vi "Loop Template.vi"() -> ()   [LabVIEW 2014]
uses:
  user.lib/_NEVSTOP/Communicable State Machine(CSM)/_Support/Priority Queue/Priority Queue.lvclass/Priority Queue.ctl
  user.lib/_NEVSTOP/Communicable State Machine(CSM)/_Support/Process/CSMP-Async Call.vi
  user.lib/_NEVSTOP/Communicable State Machine(CSM)/_Support/GlobalEvent/GEvt-Generate Status Log.vi
  user.lib/_NEVSTOP/Communicable State Machine(CSM)/_Support/Process/CSMP-Broadcast.vi
  user.lib/_NEVSTOP/Communicable State Machine(CSM)/_Support/GlobalEvent/GEvt-Generate Interrupt Log.vi
  user.lib/_NEVSTOP/Communicable State Machine(CSM)/_Support/GlobalEvent/GEvt-Generate Register Log.vi
  user.lib/_NEVSTOP/Communicable State Machine(CSM)/_Support/Process/CSMP-Register Status.vi
  user.lib/_NEVSTOP/Communicable State Machine(CSM)/_Support/GlobalEvent/GEvt-Generate Unregister Log.vi
  user.lib/_NEVSTOP/Communicable State Machine(CSM)/_Support/Process/CSMP-Unregister Status.vi
  user.lib/_NEVSTOP/Communicable State Machine(CSM)/_Support/Process/CSMP-Sync Call.vi
  user.lib/_NEVSTOP/Communicable State Machine(CSM)/_Support/CSMQ/_CSMObj-Unlock.vi
  user.lib/_NEVSTOP/Communicable State Machine(CSM)/_Support/Process/CSMP-PostPostMsg.vi
  user.lib/_NEVSTOP/Communicable State Machine(CSM)/_Support/Process/CSMP-PostSendMsg.vi
  user.lib/_NEVSTOP/Communicable State Machine(CSM)/_Support/CSMQ/_CSMObj-Lock State.vi
  user.lib/_NEVSTOP/Communicable State Machine(CSM)/_Support/Common/Splite Reason String Part.vi
  user.lib/_NEVSTOP/Communicable State Machine(CSM)/_Support/Common/Trim Single line Text.vi
  user.lib/_NEVSTOP/Communicable State Machine(CSM)/_Support/CSMQ/_CSMOFGV Release.vi
  user.lib/_NEVSTOP/Communicable State Machine(CSM)/_Support/Common/Remove Comments from Line.vi
  user.lib/_NEVSTOP/Communicable State Machine(CSM)/_Support/Common/Splite Single-line Message.vi
  user.lib/_NEVSTOP/Communicable State Machine(CSM)/_Support/Common/Parse Next Single-line State.vi
  user.lib/_NEVSTOP/Communicable State Machine(CSM)/_Support/CSMQ/_CSMOFGV Dequeue.vi
  user.lib/_NEVSTOP/Communicable State Machine(CSM)/_Support/CSMQ/_CSMObj-Log Error if in a Remote Session.vi
  user.lib/_NEVSTOP/Communicable State Machine(CSM)/_Support/GlobalEvent/GEvt-Generate State Change Log.vi
  user.lib/_NEVSTOP/Communicable State Machine(CSM)/_Support/GlobalEvent/GEvt-Generate Remaining States Log.vi
  user.lib/_NEVSTOP/Communicable State Machine(CSM)/_Support/GlobalEvent/GEvt-Generate Module Destroyed Log.vi
  user.lib/_NEVSTOP/Communicable State Machine(CSM)/_Support/GlobalEvent/GEvt-Generate Complete Log.vi
  user.lib/_NEVSTOP/Communicable State Machine(CSM)/_Support/GlobalEvent/GEvt-Generate Module Created Log.vi
  user.lib/_NEVSTOP/Communicable State Machine(CSM)/AdvanceAPI/CSM - Revert Arguments-Safe String.vi
  user.lib/_NEVSTOP/Communicable State Machine(CSM)/AdvanceAPI/CSM - Make String Arguments Safe.vi
  user.lib/_NEVSTOP/Communicable State Machine(CSM)/_Support/CSMQ/_CSMObj-Message Check.vi
  user.lib/_NEVSTOP/Communicable State Machine(CSM)/_Support/CSMQ/_CSMObj-Enqueue Cross-Module Message.vi
  user.lib/_NEVSTOP/Communicable State Machine(CSM)/_Support/CSMQ/_CSMOFGV Get.vi
  user.lib/_NEVSTOP/Communicable State Machine(CSM)/_Support/FGV-BroadcastRegistry/Cache-Broadcast Registry Search Result.vi
  user.lib/_NEVSTOP/Communicable State Machine(CSM)/AdvanceAPI/CSM - Register Status Change.vi
  user.lib/_NEVSTOP/Communicable State Machine(CSM)/AdvanceAPI/CSM - Unregister Status Change.vi
  user.lib/_NEVSTOP/Communicable State Machine(CSM)/_Support/Common/Hex Str to U8 Data.vi
  user.lib/_NEVSTOP/Communicable State Machine(CSM)/_Support/Common/Concatenate State with Arguments.vi
  user.lib/_NEVSTOP/Communicable State Machine(CSM)/_Support/Common/U8 Data to Hex Str.vi
  user.lib/_NEVSTOP/Communicable State Machine(CSM)/_Support/Priority Queue/Dequeue Element.vi
  user.lib/_NEVSTOP/Communicable State Machine(CSM)/AdvanceAPI/CSM - Keywords.vi
  user.lib/_NEVSTOP/Communicable State Machine(CSM)/_Support/Priority Queue/Enqueue Element.vi
  user.lib/_NEVSTOP/Communicable State Machine(CSM)/Utility/Trim Both Whitespace.vi
  user.lib/_NEVSTOP/Communicable State Machine(CSM)/_Support/GlobalEvent/FGV-GlobalEventRef.vi
  user.lib/_NEVSTOP/Communicable State Machine(CSM)/_Support/CSMQ/_CSMOFGV Obtain.vi
  user.lib/_NEVSTOP/Communicable State Machine(CSM)/_Support/CSMQ/_CSMOFGV.vi
  user.lib/_NEVSTOP/Communicable State Machine(CSM)/_Support/GlobalEvent/FGV-StatusChangeEventRef.vi
  user.lib/_NEVSTOP/Communicable State Machine(CSM)/_Support/FGV-BroadcastRegistry/global-Broadcast Cache Change Flag.vi
  user.lib/_NEVSTOP/Communicable State Machine(CSM)/_Support/FGV-BroadcastRegistry/FGV-BroadcastRegistry.vi
  user.lib/_NEVSTOP/Communicable State Machine(CSM)/Communicable State Machine.lvlib
  user.lib/_NEVSTOP/Communicable State Machine(CSM)/addons/Loop-Support/CSM Loop Support.lvlib
panel:
  out "Filtered UI States":string
  out "UI States":string
  out ">> Source CSM >>":string
  out "Remaining States":string
  in  "DAQ: Once":bool
  out "Waveform Chart":dbl(graph)=7.7472539242125515
  in  "Center":dbl(slide) scale=0.0..10.0
  in  "Stop":bool
  in  "Start":bool
  out "State History":string
  in  "Name(\"\" to use uuid)":string="CSM Tiny"
  in  "Init State(\"Macro: Initialize\")":string="Macro: Initialize"
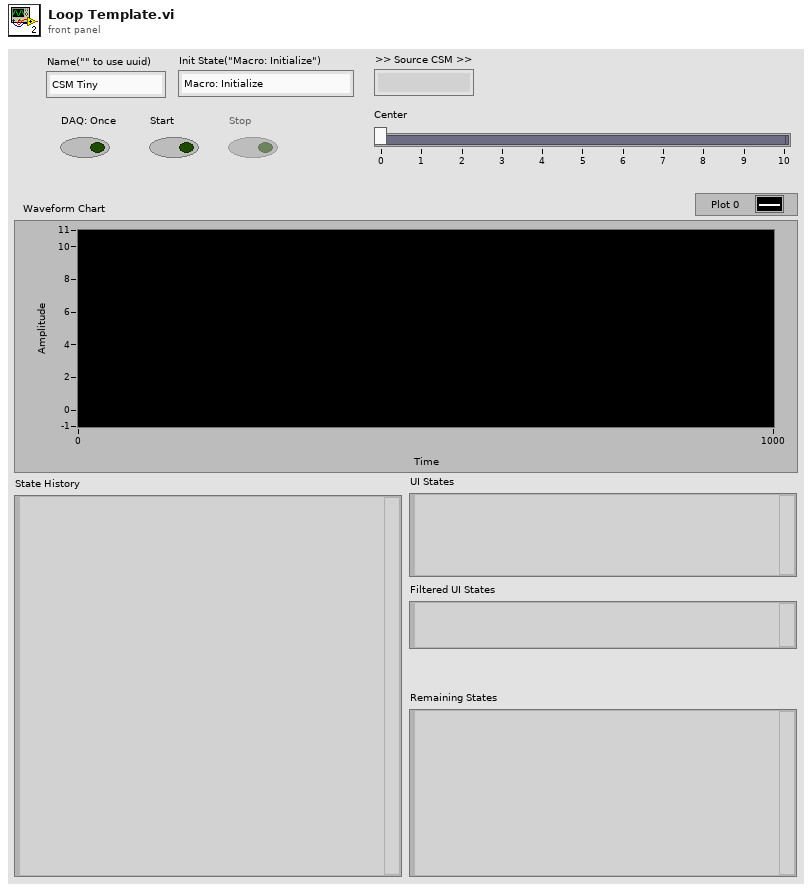
[diagram p1: front panel]
types:
  T1 = enum32{"Invalid", "Standard", "Closed", "Hidden", "Minimized", "Maximized"}
  T2 = enum32{"invalid app kind", "Development System", "Run Time System", "Student Edition", "Embedded LabVIEW", "Evaluation", "Custom"}
  T3 = typedef "Communicable State Machine.lvlib/_CSM_Response Source Message.ctl" = cluster{"‘State":string, "’Arguments":string, "’Error":errorcluster}
  T4 = cluster{"Core":cluster{"Current VI Reference":refnum<vi>, "Close Panel on Exit?":bool}, "IsRunning?":bool, "Center":dbl}
  T5 = cluster{"Current VI Reference":refnum<vi>, "Close Panel on Exit?":bool}
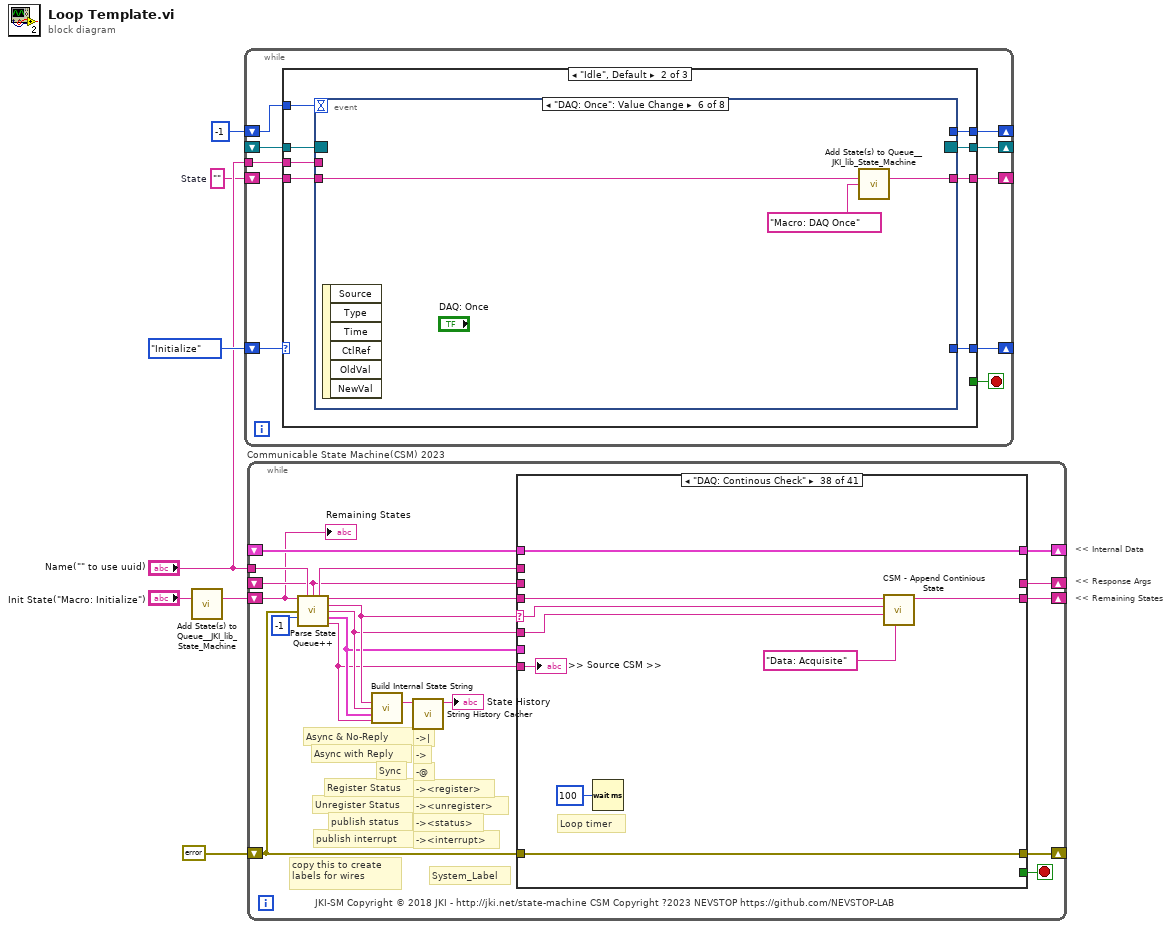
[diagram p0: block diagram]
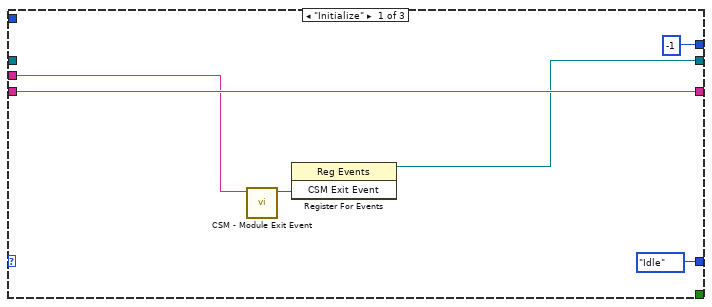
[diagram p2: hidden frame]
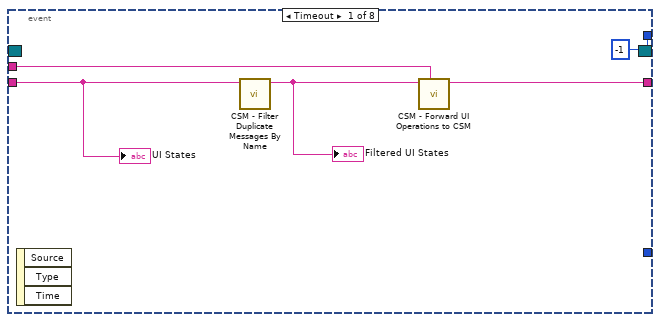
[diagram p3: hidden frame]
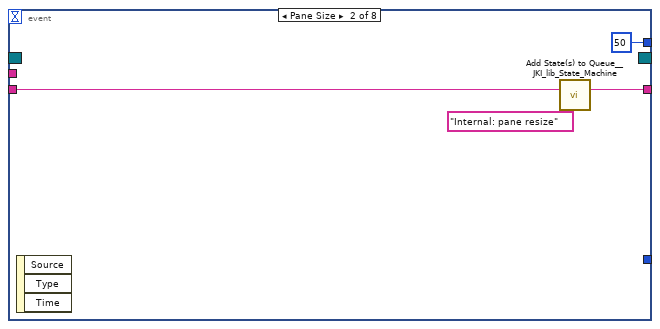
[diagram p4: hidden frame]
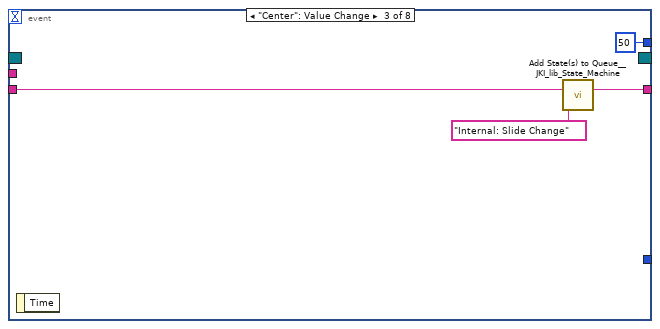
[diagram p5: hidden frame]
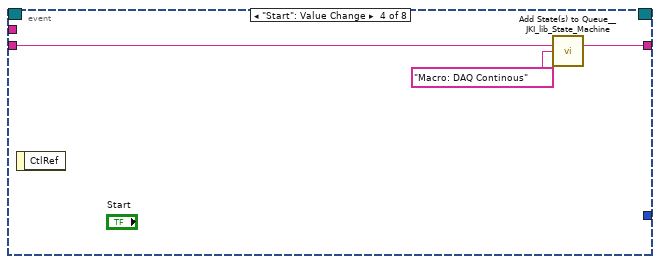
[diagram p6: hidden frame]
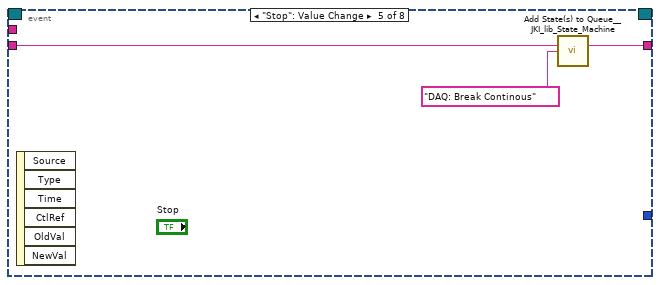
[diagram p7: hidden frame]
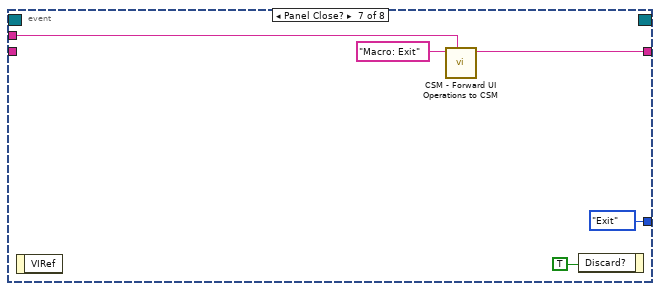
[diagram p8: hidden frame]
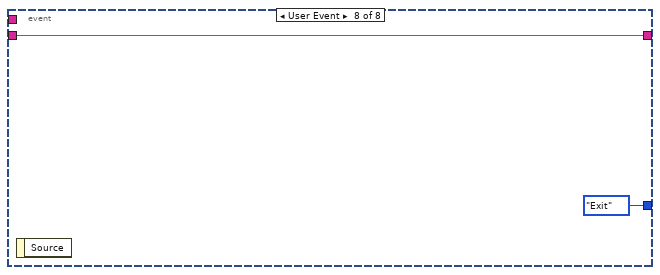
[diagram p9: hidden frame]
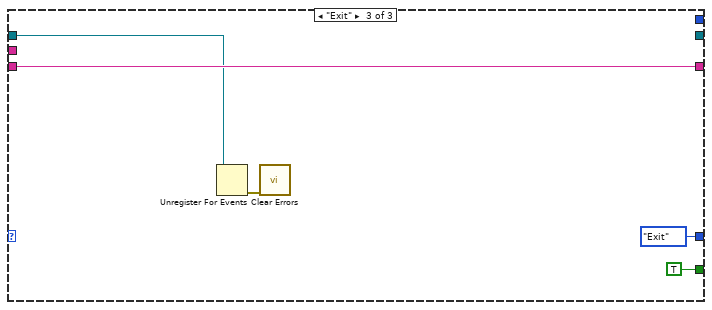
[diagram p10: hidden frame]
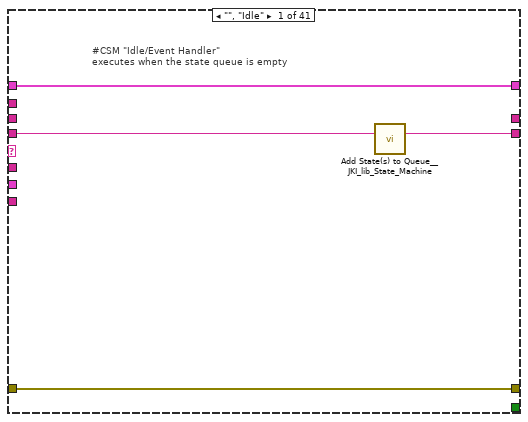
[diagram p11: hidden frame]
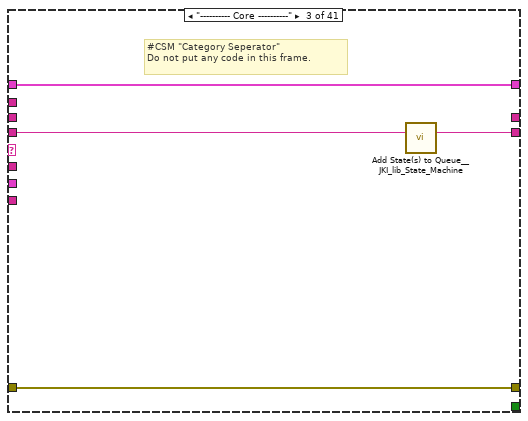
[diagram p13: hidden frame]
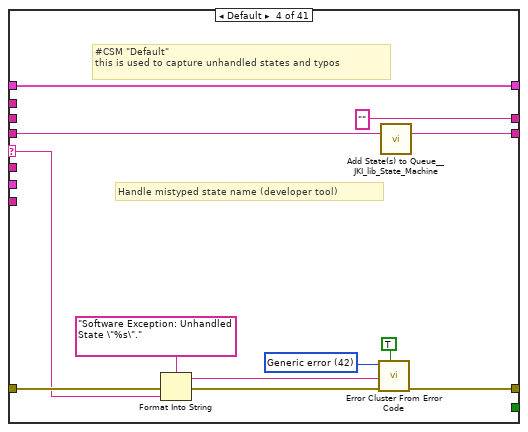
[diagram p14: hidden frame]
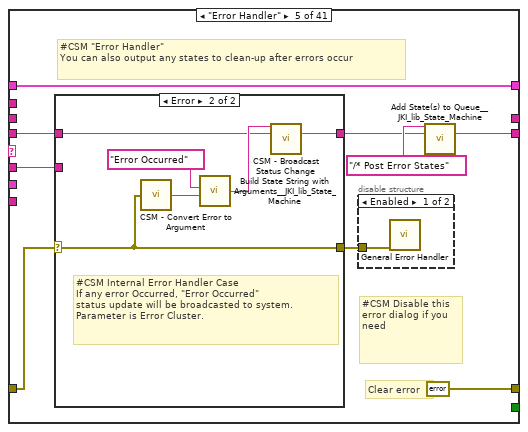
[diagram p15: hidden frame]
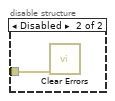
[diagram p16: hidden frame]
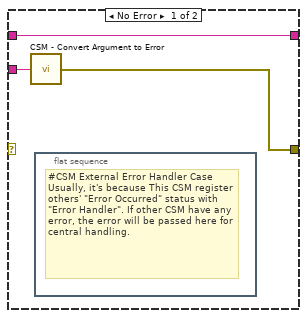
[diagram p17: hidden frame]
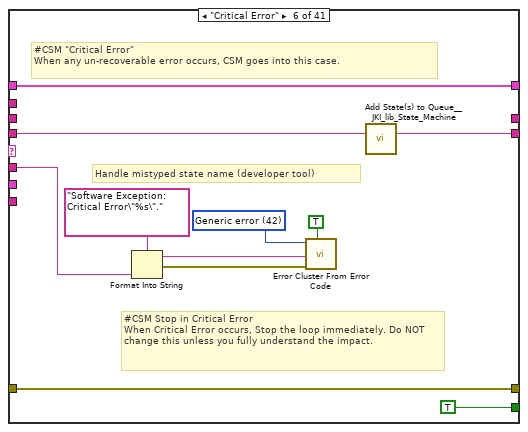
[diagram p18: hidden frame]
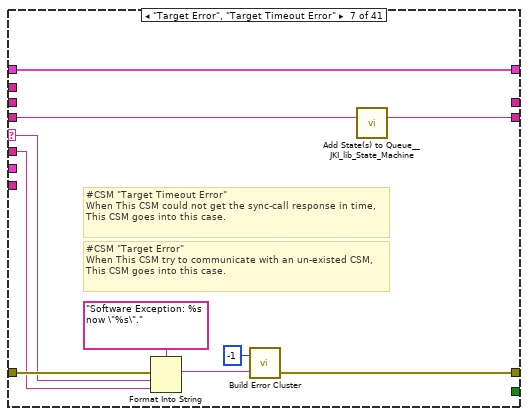
[diagram p19: hidden frame]
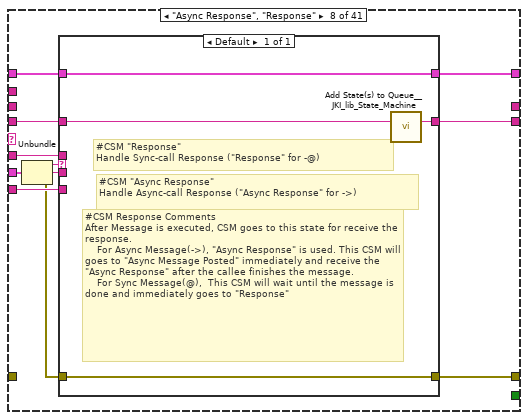
[diagram p20: hidden frame]
diagram:
  w2 = ""  # State
  # "<< Internal Data"
  # "<< Response Args"
  # "<< Remaining States"
  n1 = call <vilib>:"Add State(s) to Queue__JKI_lib_State_Machine.vi"("State(s) in (\"\")"="Init State(\"Macro: Initialize\")") -> ("States Out"=w5:string)  [unwired: 14 in]
  n2 = while {
    shift-right: [w16] -> _
    shift-left: enum16{"Idle", "Initialize", "Exit"}."Initialize" -> [w17]
    tunnel: "Name(\"\" to use uuid)" -> [w14]
    shift-right: [w12] -> _
    shift-left: w2 -> [w13]
    shift-right: [w10] -> _
    shift-left: -1 -> [w11]
    shift-right: [w9] -> _
    shift-left: _ -> [w8]
    stop <- w15 stop-if-true
    n3 = case shown="\"Idle\", Default" w17 {
      tunnel: [enum16{"Idle", "Initialize", "Exit"}."Idle" w31 enum16{"Idle", "Initialize", "Exit"}."Exit"] -> w16
      tunnel: [_ _ TRUE] -> w15
      tunnel: w14 -> [w19 w30 _]
      tunnel: w13 -> [w22 w28 w63]
      tunnel: [w22 w29 w63] -> w12
      tunnel: w11 -> [_ w26 _]
      tunnel: [-1 w27 _] -> w10
      tunnel: [w18 w24 _] -> w9
      tunnel: w8 -> [_ w25 w62]
      frame "Initialize" {
        n4 = call "CSM - Module Exit Event.vi"("Name(\"\" to use uuid) in"=w19) -> ("CSM Exit Event"=w20:refnum<user-event>)  [unwired: 9 in, 1 out]
        n5 = register-events(w20) -> (reference out=w18:refnum<event-registration>)  [unwired: 2 in, 1 out]
      }
      frame "Idle", Default {
        n6 = event shown="[5] \"DAQ: Once\": Value Change" {
          selector: w25 -> [_ _ _ _ _ _ _ _]
          dyn-events: [_ _ _ _ _ _ _ _] -> w24
          timeout: w26 -> [_ _ _ _ _ _ _ _]
          tunnel: [_ _ _ _ _ _ enum16{"Idle", "Initialize", "Exit"}."Exit" enum16{"Idle", "Initialize", "Exit"}."Exit"] -> w31
          tunnel: w30 -> [w32 _ _ _ _ _ w55 _]
          tunnel: w28 -> [w35 w40 w44 w47 w49 w52 _ w60]
          tunnel: [w33 w39 w43 w46 w50 w53 w54 w60] -> w29
          tunnel: [-1 50 50 _ _ _ _ _] -> w27
          event Timeout {
            n7 = event-data() -> ()  [unwired: 1 in, 3 out]
            n8 = call "CSM - Filter Duplicate Messages By Name.vi"("States"=w35) -> ("States out"=w34:string)  [unwired: 10 in]
            "Filtered UI States" <- w34
            n9 = call "CSM - Forward UI Operations to CSM.vi"("Name(\"\" to use uuid)"=w32, "State(s) in (\"\")"=w34) -> ("States Out"=w33:string)  [unwired: 9 in]
            "UI States" <- w35
          }
          event Pane Size {
            n10 = event-data() -> ()  [unwired: 1 in, 3 out]
            n11 = call <vilib>:"Add State(s) to Queue__JKI_lib_State_Machine.vi"("State(s) in (\"\")"=w40, "State(s) at Back (\"\")"="Internal: pane resize" ("State(s) at Back (\"\")")) -> ("States Out"=w39:string)  [unwired: 13 in]
          }
          event "Center": Value Change {
            n12 = event-data() -> ()  [unwired: 1 in, 1 out]
            n13 = call <vilib>:"Add State(s) to Queue__JKI_lib_State_Machine.vi"("State(s) in (\"\")"=w44, "State(s) at Back (\"\")"="Internal: Slide Change" ("State(s) at Back (\"\")")) -> ("States Out"=w43:string)  [unwired: 13 in]
          }
          event "Start": Value Change {
            n14 = event-data() -> ()  [unwired: 1 in, 1 out]
            n15 = call <vilib>:"Add State(s) to Queue__JKI_lib_State_Machine.vi"("State(s) in (\"\")"=w47, "State(s) at Back (\"\")"="Macro: DAQ Continous" ("State(s) at Back (\"\")")) -> ("States Out"=w46:string)  [unwired: 13 in]
          }
          event "Stop": Value Change {
            n16 = event-data() -> ()  [unwired: 1 in, 6 out]
            n17 = call <vilib>:"Add State(s) to Queue__JKI_lib_State_Machine.vi"("State(s) in (\"\")"=w49, "State(s) at Back (\"\")"="DAQ: Break Continous" ("State(s) at Back (\"\")")) -> ("States Out"=w50:string)  [unwired: 13 in]
          }
          event "DAQ: Once": Value Change {
            n18 = event-data() -> ()  [unwired: 1 in, 6 out]
            n19 = call <vilib>:"Add State(s) to Queue__JKI_lib_State_Machine.vi"("State(s) in (\"\")"=w52, "State(s) at Back (\"\")"="Macro: DAQ Once" ("State(s) at Back (\"\")")) -> ("States Out"=w53:string)  [unwired: 13 in]
          }
          event Panel Close? {
            n20 = event-data() -> ()  [unwired: 1 in, 1 out]
            n21 = call "CSM - Forward UI Operations to CSM.vi"("Name(\"\" to use uuid)"=w55, "State(s) in (\"\")"="Macro: Exit" ("State")) -> ("States Out"=w54:string)  [unwired: 9 in]
            n22 = event-data("Discard?"=TRUE) -> ()  [unwired: 1 in, 1 out]
          }
          event User Event {
            n23 = event-data() -> ()  [unwired: 1 in, 1 out]
          }
        }
      }
      frame "Exit" {
        n24 = Unregister For Events(event registration refnum=w62) -> (error out=w61:errorcluster)  [unwired: 1 in]
        n25 = call <vilib>:"Clear Errors.vi"("error in (no error)"=w61) -> ()  [unwired: 5 in, 2 out]
      }
    }
  }
  n26 = while "Communicable State Machine(CSM) 2023" {
    shift-right: [w80] -> _
    shift-left: _ -> [w79]
    shift-right: [w83] -> _
    shift-left: errorcluster {"status"=FALSE, "code"=0, "source"=""} ("error out") -> [w78]
    shift-right: [w82] -> _
    shift-left: w5 -> [w66]
    tunnel: "Name(\"\" to use uuid)" -> [w76]
    shift-right: [w77] -> _
    shift-left: _ -> [w68]
    stop <- w81 stop-if-true
    # "-><interrupt>"
    # "-><status>"
    # "-><unregister>"
    # "-><register>"
    # "-@"
    # "->"
    # "->|"
    # "publish interrupt"
    # "publish status"
    # "Unregister Status"
    # "Register Status"
    # "Sync"
    # "Async with Reply"
    # "Async & No-Reply"
    # "copy this to create labels for wires"
    # "System_Label"
    # "JKI-SM Copyright © 2018 JKI - http://jki.net/state-machine CSM Copyright ?2023 NEVSTOP https://github.com/NEVSTOP-LAB"
    n27 = call "Parse State Queue++.vi"("State Queue"=w66, "Name(\"\" to use uuid)"=w76, "Response Arguments"=w68, "Error In (no error)"=w78, "Dequeue Timeout(0ms)"=-1 ("Timeout")) -> ("Name Used"=w69:string, "Remaining States"=w84:string, "Current State"=w73:string, "Arguments"=w72:string, ">> Response Source Message >>"=w71:T3, ">> Source CSM >>"=w70:string)  [unwired: 5 in]
    n28 = call "Build Internal State String.vi"("State"=w73, "Arguments (\"\")"=w72, ">> Response Source Message >>"=w71, "Source (\"\")"=w70) -> ("State with Arguments"=w74:string)  [unwired: 11 in]
    n29 = call "String History Cacher.vi"("String"=w74) -> ("String Cache"=→"State History":string)  [unwired: 10 in]
    n30 = case shown="\"DAQ: Continous Check\"" w73 {
      selector: w73 -> [_ _ _ w97 _ _ w142 _ _ _ _ _ _ _ _ _ _ _ _ _ _ _ _ _ _ _ _ _ _ _ _ _ _ _ _ _ _ w394 _ _ _]
      tunnel: w84 -> [w85 w90 w95 w101 w112 w136 w144 w154 w165 w179 w184 w188 w195 w197 w204 w208 w214 w220 w235 w313 w318 w323 w325 w330 w334 w342 w346 w351 w358 w362 w366 w370 w373 w376 w379 w384 w390 w396 w402 w408 w411]
      tunnel: w72 -> [_ _ _ _ w111 w129 w143 w153 _ _ _ _ _ _ _ _ _ w215 w229 _ _ _ _ _ _ _ _ w349 _ _ _ _ _ _ _ _ _ w393 _ _ _]
      tunnel: w79 -> [w86 w89 w92 w99 w115 w137 w145 w156 w164 w172 w182 w185 _ w196 w199 w205 w212 w218 w231 w312 w315 w320 w327 w332 w336 w341 w345 w350 w355 w359 w363 w369 w372 w375 w378 w383 w387 w399 w403 w407 w410]
      tunnel: [w87 w91 w93 w103 errorcluster {"status"=FALSE, "code"=0, "source"=""} ("error out") w138 w140 w159 w166 w176 w181 w186 w192 w198 w200 w206 w211 w216 w232 w314 w316 w321 w328 w333 w339 w343 w347 w352 w356 w360 w364 w371 w374 w377 w380 w385 w391 w400 w404 w409 w412] -> w83
      tunnel: w78 -> [w87 w91 w93 w102 w113 w138 w147 _ w166 w176 w181 w186 w192 w198 w201 w206 w211 w217 w233 w314 w316 w321 w328 w333 w339 w343 w347 w352 w356 w360 w364 w371 w374 w377 w380 w385 w391 w400 w404 w409 w412]
      tunnel: [w88 w90 w94 w100 w108 w135 w146 w155 w165 w178 w183 w187 w194 w197 w203 w207 w213 w219 w234 w313 w317 w322 w326 w331 w340 w342 w346 w351 w357 w361 w365 w370 w373 w376 w379 w384 w390 w397 w401 w408 w411] -> w82
      tunnel: [_ _ _ _ _ TRUE _ _ _ _ TRUE _ _ _ _ _ _ _ _ _ _ _ _ _ _ _ _ _ _ _ _ _ _ _ _ _ _ _ _ _ _] -> w81
      tunnel: [w86 w89 w92 w99 w115 w137 w145 w157 w164 w177 w182 w185 w193 w196 w199 w205 w212 w218 w231 w312 w315 w320 w327 w332 w336 w341 w345 w350 w355 w359 w363 w368 w372 w375 w378 w382 w387 w399 w403 w406 w410] -> w80
      tunnel: w70 -> [_ _ _ _ _ _ _ w151 _ _ _ _ _ _ _ _ _ _ _ _ _ _ _ _ _ _ _ _ _ _ _ _ _ _ _ _ _ w395 _ _ _]
      tunnel: w71 -> [_ _ _ _ _ _ _ w158 _ _ _ _ _ _ _ _ _ _ _ _ _ _ _ _ _ _ _ _ _ _ _ _ _ _ _ _ _ _ _ _ _]
      tunnel: [_ _ _ "" _ _ _ _ _ _ _ _ _ _ _ _ _ _ _ _ _ _ _ _ _ _ "API1 Response" w348 _ _ _ _ _ _ _ _ _ _ _ _ _] -> w77
      tunnel: w69 -> [_ _ _ _ _ _ _ _ _ _ _ _ _ _ _ _ _ _ _ _ _ _ _ _ _ _ _ _ _ _ _ _ _ _ _ _ _ _ _ _ _]
      tunnel: w68 -> [_ _ _ _ _ _ _ _ _ _ _ _ _ _ _ _ _ _ _ _ _ _ _ _ _ _ _ _ _ _ _ _ _ _ _ _ _ _ _ _ _]
      frame "", "Idle" {
        # "#CSM \"Idle/Event Handler\"\nexecutes when the state queue is empty"
        n31 = call <vilib>:"Add State(s) to Queue__JKI_lib_State_Machine.vi"("State(s) in (\"\")"=w85) -> ("States Out"=w88:string)  [unwired: 14 in]
      }
      frame "CSM Documentation" {
        # "#CSM README FIRST\n\nCSM is a LabVIEW application framework that builds upon JKI State Machine (JKISM). It follows the pattern of JKISM and extends the keywords to describe message communication between CSM modules, including concepts such as Sync-Message, Async-Message, Subscription/Unsubscription of status - essential elements for creating reusable code modules. For more information, please visit the CSM wiki: https://github.com/NEVSTOP-LAB/JKI-State-Machine-Plus-Plus/wiki\n\nFor instructions on JKI State Machine, visit: http://jki.net/state-machine/\nFor information about CSM, visit: https://github.com/NEVSTOP-LAB"
        # "#CSM \"Documentation\"\nCase for holding CSM Documenation"
      }
      frame "---------- Core ----------" {
        # "#CSM \"Category Seperator\"\nDo not put any code in this frame."
        n32 = call <vilib>:"Add State(s) to Queue__JKI_lib_State_Machine.vi"("State(s) in (\"\")"=w95) -> ("States Out"=w94:string)  [unwired: 14 in]
      }
      frame Default {
        w106 = 42 items=["No error", "Argument error", "Memory is full", "Out of zone", "End of file", "File already open", "Generic file I/O error", "File not found", "File permission error", "Disk is full", "Duplicate path", "Too many files open", "System feature not enabled", "Resource file not found", "Cannot add resource", "Resource not found", "Image not found", "Image memory error", "Pen does not exist", "Config type invalid", "Config token not found", "Config parse error", "Config memory error", "Bad external code format", "Bad external code offset", "External code not present", "Null window", "Destroy window error", "Null menu", "Print aborted", "Bad print record", "Print driver error", "Windows error during printing", "Memory error during printing", "Print dialog error", "Generic print error", "Invalid device refnum", "Device not found", "Device parameter error", "Device unit error", "Cannot open device", "Device call aborted", "Generic error", "Cancelled by user", "Object ID too low", "Object ID too high", "Object not in heap", "Unknown heap", "Unknown object (invalid DefProc)", "Unknown object (DefProc not in table)", "Message out of range", "Invalid (null) method", "Unknown message", "Manager call not supported", "Bad address", "Network operation in progress", "Network operation timed out", "Connection is busy", "Network attribute not supported", "Network error", "Address in use", "System out of memory", "Connection aborted", "Connection refused", "Not connected", "Already connected", "Connection closed", "Initialization error (interapplication manager)", "Bad occurrence", "Wait on unbound occurrence handler", "Occurrence queue overflow", "Datalog type conflict", "Unused", "Unrecognized type (interapplication manager)", "Memory corrupt", "Failed to make temporary DLL", "Old CIN version", "Drag socket not found", "Failed to load drop-object", "Failed to register OLE object", "Failed to release OLE object", "Format specifier type mismatch", "Unknown format specifier", "Too few format specifiers", "Too many format specifiers", "Scan failed", "Newer CIN version", "Error converting to variant", "Runtime menu error", "Password tampered", "Variant attribute not found", "Incompatible variant data type", "Event data is not available", "Event Store is not present", "Occurrence is not found", "Event Queue is not created", "Event info is not available", "Refnum passed is NULL", "Error retrieving Class GUID", "Error retrieving CoClass GUID", "Error retrieving TypeLib GUID.", "Bad built application magic bytes.", "Specific driver is different from the specific driver associated with the Logical Name.", "There is no session opened to the class driver.", "Max Error", "MAX - Error with config objects", "MAX - Error loading configuration", "MAX - Group not supported"]
        # "#CSM \"Default\"\nthis is used to capture unhandled states and typos"
        # "Handle mistyped state name (developer tool)"
        n33 = Format Into String(format string="Software Exception: Unhandled State \"%s\"." ("message"), error in=w102, w97) -> (resulting string=w105:string, error out=w104:errorcluster)  [unwired: 1 in]
        n34 = call <vilib>:"Error Cluster From Error Code.vi"("show call chain? (False)"=TRUE, "error in (no error)"=w104, "error message (\"\")"=w105, "error code (0)"=w106) -> ("error out"=w103:errorcluster)  [unwired: 5 in]
        n35 = call <vilib>:"Add State(s) to Queue__JKI_lib_State_Machine.vi"("State(s) in (\"\")"=w101) -> ("States Out"=w100:string)  [unwired: 14 in]
      }
      frame "Error Handler" {
        # "#CSM Disable this error dialog if you need"
        # "#CSM \"Error Handler\"\nYou can also output any states to clean-up after errors occur"
        # "Clear error"
        n36 = case shown="Error" w113 {
          selector: w113 -> [_ w122]
          tunnel: [w121 w124] -> w109
          tunnel: w112 -> [w121 w123]
          tunnel: w111 -> [w120 _]
          tunnel: [w119 w122] -> w114
          frame No Error {
            n37 = call "CSM - Convert Argument to Error.vi"("Argument"=w120) -> ("error"=w119:errorcluster)  [unwired: 4 in]
            n38 = flat-sequence {
              frame #0 {
                # "#CSM External Error Handler Case\nUsually, it's because This CSM register others' \"Error Occurred\" status with \"Error Handler\". If other CSM have any error, the error will be passed here for central handling."
              }
            }
          }
          frame Error {
            # "#CSM Internal Error Handler Case \nIf any error Occurred, \"Error Occurred\" \nstatus update will be broadcasted to system.\nParameter is Error Cluster."
            n39 = call "CSM - Convert Error to Argument.vi"("error in (no error)"=w122) -> ("Arguments"=w126:string)  [unwired: 4 in]
            n40 = call <vilib>:"Build State String with Arguments__JKI_lib_State_Machine.vi"("Arguments (\"\")"=w126, "State"="Error Occurred" ("Status with Arguments")) -> ("State with Arguments"=w125:string)  [unwired: 4 in]
            n41 = call "CSM - Broadcast Status Change.vi"("Status with Arguments"=w125, "State Queue"=w123) -> ("Remaining States"=w124:string)  [unwired: 13 in]
          }
        }
        n42 = disable-structure shown="Enabled" {
          disable-tunnel: w114 -> [w117 w118]
          frame Enabled {
            n43 = call <vilib>:"General Error Handler.vi"("error in (no error)"=w117) -> ()  [unwired: 10 in, 5 out]
          }
          frame Disabled {
            n44 = call <vilib>:"Clear Errors.vi"("error in (no error)"=w118) -> ()  [unwired: 5 in, 2 out]
          }
        }
        n45 = call <vilib>:"Add State(s) to Queue__JKI_lib_State_Machine.vi"("State(s) in Front (\"\")"="/* Post Error States", "State(s) in (\"\")"=w109) -> ("States Out"=w108:string)  [unwired: 13 in]
      }
      frame "Critical Error" {
        w133 = 42 items=["No error", "Argument error", "Memory is full", "Out of zone", "End of file", "File already open", "Generic file I/O error", "File not found", "File permission error", "Disk is full", "Duplicate path", "Too many files open", "System feature not enabled", "Resource file not found", "Cannot add resource", "Resource not found", "Image not found", "Image memory error", "Pen does not exist", "Config type invalid", "Config token not found", "Config parse error", "Config memory error", "Bad external code format", "Bad external code offset", "External code not present", "Null window", "Destroy window error", "Null menu", "Print aborted", "Bad print record", "Print driver error", "Windows error during printing", "Memory error during printing", "Print dialog error", "Generic print error", "Invalid device refnum", "Device not found", "Device parameter error", "Device unit error", "Cannot open device", "Device call aborted", "Generic error", "Cancelled by user", "Object ID too low", "Object ID too high", "Object not in heap", "Unknown heap", "Unknown object (invalid DefProc)", "Unknown object (DefProc not in table)", "Message out of range", "Invalid (null) method", "Unknown message", "Manager call not supported", "Bad address", "Network operation in progress", "Network operation timed out", "Connection is busy", "Network attribute not supported", "Network error", "Address in use", "System out of memory", "Connection aborted", "Connection refused", "Not connected", "Already connected", "Connection closed", "Initialization error (interapplication manager)", "Bad occurrence", "Wait on unbound occurrence handler", "Occurrence queue overflow", "Datalog type conflict", "Unused", "Unrecognized type (interapplication manager)", "Memory corrupt", "Failed to make temporary DLL", "Old CIN version", "Drag socket not found", "Failed to load drop-object", "Failed to register OLE object", "Failed to release OLE object", "Format specifier type mismatch", "Unknown format specifier", "Too few format specifiers", "Too many format specifiers", "Scan failed", "Newer CIN version", "Error converting to variant", "Runtime menu error", "Password tampered", "Variant attribute not found", "Incompatible variant data type", "Event data is not available", "Event Store is not present", "Occurrence is not found", "Event Queue is not created", "Event info is not available", "Refnum passed is NULL", "Error retrieving Class GUID", "Error retrieving CoClass GUID", "Error retrieving TypeLib GUID.", "Bad built application magic bytes.", "Specific driver is different from the specific driver associated with the Logical Name.", "There is no session opened to the class driver.", "Max Error", "MAX - Error with config objects", "MAX - Error loading configuration", "MAX - Group not supported"]
        # "#CSM Stop in Critical Error\nWhen Critical Error occurs, Stop the loop immediately. Do NOT change this unless you fully understand the impact."
        # "#CSM \"Critical Error\"\nWhen any un-recoverable error occurs, CSM goes into this case."
        # "Handle mistyped state name (developer tool)"
        n46 = Format Into String(format string="Software Exception: Critical Error\"%s\"." ("message"), w129) -> (resulting string=w132:string, error out=w131:errorcluster)  [unwired: 2 in]
        n47 = call <vilib>:"Error Cluster From Error Code.vi"("show call chain? (False)"=TRUE, "error in (no error)"=w131, "error message (\"\")"=w132, "error code (0)"=w133) -> ()  [unwired: 5 in, 1 out]
        n48 = call <vilib>:"Add State(s) to Queue__JKI_lib_State_Machine.vi"("State(s) in (\"\")"=w136) -> ("States Out"=w135:string)  [unwired: 14 in]
      }
      frame "Target Error", "Target Timeout Error" {
        # "#CSM \"Target Error\"\nWhen This CSM try to communicate with an un-existed CSM, This CSM goes into this case."
        # "#CSM \"Target Timeout Error\"\nWhen This CSM could not get the sync-call response in time, This CSM goes into this case."
        n49 = Format Into String(format string="Software Exception: %s now \"%s\"." ("message"), error in=w147, w142, w143) -> (resulting string=w141:string)  [unwired: 1 in, 1 out]
        n50 = call "Build Error Cluster.vi"("String to Prepend to source (\"\")"=w141, "code"=-1) -> ("error out"=w140:errorcluster)
        n51 = call <vilib>:"Add State(s) to Queue__JKI_lib_State_Machine.vi"("State(s) in (\"\")"=w144) -> ("States Out"=w146:string)  [unwired: 14 in]
      }
      frame "Async Response", "Response" {
        n52 = Unbundle(w158) -> ("‘State"=w152:string, "’Arguments"=w150:string, "’Error"=w149:errorcluster)
        n53 = case shown="Default" w152 {
          tunnel: [w163] -> w159
          tunnel: w149 -> [w163]
          tunnel: [w162] -> w157
          tunnel: w156 -> [w162]
          tunnel: [w160] -> w155
          tunnel: w154 -> [w161]
          tunnel: w153 -> [_]
          tunnel: w151 -> [_]
          tunnel: w150 -> [_]
          frame Default {
            # "#CSM Response Comments\nAfter Message is executed, CSM goes to this state for receive the response.\n    For Async Message(->), \"Async Response\" is used. This CSM will goes to \"Async Message Posted\" immediately and receive the \"Async Response\" after the callee finishes the message.\n    For Sync Message(@),  This CSM will wait until the message is done and immediately goes to \"Response\""
            # "#CSM \"Async Response\"\nHandle Async-call Response (\"Async Response\" for ->)"
            # "#CSM \"Response\"\nHandle Sync-call Response (\"Response\" for -@)"
            n54 = call <vilib>:"Add State(s) to Queue__JKI_lib_State_Machine.vi"("State(s) in (\"\")"=w161) -> ("States Out"=w160:string)  [unwired: 14 in]
          }
        }
      }
      frame "Async Message Posted" {
        # "#CSM \"Async Message Posted\"\nAfter Async Message is posted (-> or ->| ), CSM goes to this state for post-action.\nYou can use Argument - State to tell which Async Message is called."
      }
      frame "Initialize Core Data" {
        # "#CSM \"Initialize Core Data\"\nThis is used to determine panel behavior on exit"
        # "originally closed?"
        # "exe?"
        # "If panel starts closed or is an EXE, then close it when we exit"
        n55 = property class="VI"() -> ("FP.State"=w169:T1)  [unwired: 2 in, 2 out]
        n56 = property class="App"() -> ("App.Kind"=w175:T2)  [unwired: 2 in, 2 out]
        n57 = control-ref of="Current VI Reference"() -> (w170:refnum<vi>)
        n58 = Equal?(x=w169, y=T1."Closed" ("Front Panel Window:State")) -> (x = y?=w167:bool)
        n59 = Equal?(x=w175, y=T2."Run Time System" ("Application:Kind")) -> (x = y?=w173:bool)
        n60 = Or(x=w167, y=w173) -> (x .or. y?=w171:bool)
        n61 = Bundle By Name(cluster=w172, "Core.Current VI Reference"=w170, "Core.Close Panel on Exit?"=w171) -> (w177:T4)
        n62 = call <vilib>:"Add State(s) to Queue__JKI_lib_State_Machine.vi"("State(s) in (\"\")"=w179) -> ("States Out"=w178:string)  [unwired: 14 in]
      }
      frame "Exit" {
        # "#CSM \"Exit\"\nCase for exiting the loop. No errors that occur here will be handled."
        n63 = call <vilib>:"Add State(s) to Queue__JKI_lib_State_Machine.vi"("State(s) in (\"\")"=w184) -> ("States Out"=w183:string)  [unwired: 14 in]
      }
      frame "---------- Data ----------" {
        # "#CSM \"Category Seperator\"\nDo not put any code in this frame."
        n64 = call <vilib>:"Add State(s) to Queue__JKI_lib_State_Machine.vi"("State(s) in (\"\")"=w188) -> ("States Out"=w187:string)  [unwired: 14 in]
      }
      frame "Data: Initialize" {
        w190 = T5 {"Current VI Reference"=refnum, "Close Panel on Exit?"=FALSE}  # Core
        w191 = FALSE  # IsRunning?
        # "do not delete - used by framework"
        # "Expand Bundle to add new data elements to shift register data."
        # "Initialize the shift-register data, here.\n(data names are defined by what you wire into the bundle function)"
        n65 = local read "Center"() -> (w189:dbl)
        n66 = Bundle("Core"=w190, "IsRunning?"=w191, "Center"=w189) -> (w193:T4)  [unwired: 1 in]
        n67 = call <vilib>:"Add State(s) to Queue__JKI_lib_State_Machine.vi"("State(s) in (\"\")"=w195) -> ("States Out"=w194:string)  [unwired: 14 in]
      }
      frame "Data: Update Indicators" {
      }
      frame "Data: Cleanup" {
        # "Cleanup any data and references, here.\n(this is called automatically, by the Macro: Exit)"
        n68 = Unbundle By Name(w199) -> ("Core.Current VI Reference"=w202:refnum<vi>)
        n69 = Close Reference(reference=w202, error in (no error)=w201) -> (error out=w200:errorcluster)
        n70 = call <vilib>:"Add State(s) to Queue__JKI_lib_State_Machine.vi"("State(s) in (\"\")"=w204) -> ("States Out"=w203:string)  [unwired: 14 in]
      }
      frame "---------- UI ----------" {
        # "#CSM \"Category Seperator\"\nDo not put any code in this frame."
        n71 = call <vilib>:"Add State(s) to Queue__JKI_lib_State_Machine.vi"("State(s) in (\"\")"=w208) -> ("States Out"=w207:string)  [unwired: 14 in]
      }
      frame "UI: Initialize" {
        # "#CSM \"UI: Initialize\"\nInitialize the User Interface, here.\n(this is called automatically, by the Macro: Init)"
        n72 = property on="Waveform Chart" class="WFChart (strict)"("History Data"=dbl[] []) -> ()  [unwired: 2 in, 2 out]
        n73 = call <vilib>:"Add State(s) to Queue__JKI_lib_State_Machine.vi"("State(s) in Front (\"\")"="UI: Refresh Buttons" ("State(s) in Front (\"\")"), "State(s) in (\"\")"=w214) -> ("States Out"=w213:string)  [unwired: 13 in]
      }
      frame "UI: Cursor Set" {
        # "#CSM \"UI: Cursor Set\"\nSet and Unset Cursor Busy.\n(Usage: \"UI: Cursor Set >> Busy|Idle\")"
        # "Argument"
        n74 = disable-structure shown="TARGET_TYPE!=Windows" {
          disable-tunnel: w217 -> [w223 w228]
          disable-tunnel: [w222 w228] -> w216
          disable-tunnel: w215 -> [w221 _]
          frame condition #0 (active) {
            n75 = case shown="\"Idle\", Default" w221 {
              tunnel: w223 -> [w225 w227]
              tunnel: [w224 w226] -> w222
              frame "Idle", Default {
                n76 = call <vilib>:"Unset Busy.vi"("error in (no error)"=w225) -> ("error out"=w224:errorcluster)  [unwired: 10 in]
              }
              frame "Busy" {
                n77 = call <vilib>:"Set Busy.vi"("error in (no error)"=w227) -> ("error out"=w226:errorcluster)  [unwired: 9 in, 1 out]
              }
            }
          }
          frame condition #1 {
          }
        }
        n78 = call <vilib>:"Add State(s) to Queue__JKI_lib_State_Machine.vi"("State(s) in (\"\")"=w220) -> ("States Out"=w219:string)  [unwired: 14 in]
      }
      frame "UI: Front Panel State" {
        # "#CSM \"UI: Front Panel State\"\nSet Front Panel Open or Closed\n(Usage: \"UI: Front Panel State >> Open|Close\")"
        # "Argument"
        n79 = Unbundle By Name(w231) -> ("Core.Current VI Reference"=w230:refnum<vi>)
        n80 = call <vilib>:"Add State(s) to Queue__JKI_lib_State_Machine.vi"("State(s) in (\"\")"=w235) -> ("States Out"=w234:string)  [unwired: 14 in]
        n81 = case shown="\"Close\", \"Closed\"" w229 {
          tunnel: w233 -> [w241 w256 w267 w280 w293]
          tunnel: [w243 w257 w269 w282 w295] -> w232
          tunnel: w230 -> [w242 w254 w268 w281 w294]
          frame "Open", "Standard", Default {
            w236 = T1."Standard" ("State")
            n82 = property class="VI"(reference=w242, error in=w241) -> (reference out=w239:refnum<vi>, error out=w240:errorcluster, "FP.State"=w238:T1)
            n83 = Not Equal?(x=w238, y=w236) -> (x != y?=w237:bool)
            n84 = case shown="True" w237 {
              tunnel: [w247 w249] -> w243
              tunnel: w240 -> [w246 w249]
              tunnel: w239 -> [w245 _]
              tunnel: w236 -> [w244 _]
              frame True {
                n85 = invoke class="VI" method="FP.Open"(reference=w245, error in=w246, "Activate"=TRUE, "State"=w244) -> (error out=w247:errorcluster)  [unwired: 1 in, 4 out]
              }
              frame False {
              }
            }
          }
          frame "Close", "Closed" {
            n86 = property class="VI"(reference=w254, error in=w256) -> (reference out=w253:refnum<vi>, error out=w255:errorcluster, "FP.State"=w251:T1)
            n87 = Not Equal?(x=w251, y=T1."Closed" ("Front Panel Window:State")) -> (x != y?=w250:bool)
            n88 = case shown="False" w250 {
              tunnel: [w258 w261] -> w257
              tunnel: w255 -> [w258 w260]
              tunnel: w253 -> [_ w259]
              frame False {
              }
              frame True {
                n89 = invoke class="VI" method="FP.Close"(reference=w259, error in=w260) -> (error out=w261:errorcluster)  [unwired: 1 in, 2 out]
              }
            }
          }
          frame "Hidden", "Hide" {
            w262 = T1."Hidden" ("State")
            n90 = property class="VI"(reference=w268, error in=w267) -> (reference out=w265:refnum<vi>, error out=w266:errorcluster, "FP.State"=w264:T1)
            n91 = Not Equal?(x=w264, y=w262) -> (x != y?=w263:bool)
            n92 = case shown="True" w263 {
              tunnel: [w273 w274] -> w269
              tunnel: w266 -> [w272 w274]
              tunnel: w265 -> [w271 _]
              tunnel: w262 -> [w270 _]
              frame True {
                n93 = invoke class="VI" method="FP.Open"(reference=w271, error in=w272, "State"=w270) -> (error out=w273:errorcluster)  [unwired: 2 in, 4 out]
              }
              frame False {
              }
            }
          }
          frame "Minimize", "Minimized" {
            w275 = T1."Minimized" ("State")
            n94 = property class="VI"(reference=w281, error in=w280) -> (reference out=w278:refnum<vi>, error out=w279:errorcluster, "FP.State"=w277:T1)
            n95 = Not Equal?(x=w277, y=w275) -> (x != y?=w276:bool)
            n96 = case shown="True" w276 {
              tunnel: [w286 w287] -> w282
              tunnel: w279 -> [w285 w287]
              tunnel: w278 -> [w284 _]
              tunnel: w275 -> [w283 _]
              frame True {
                n97 = invoke class="VI" method="FP.Open"(reference=w284, error in=w285, "State"=w283) -> (error out=w286:errorcluster)  [unwired: 2 in, 4 out]
              }
              frame False {
              }
            }
          }
          frame "Maximize", "Maximized" {
            w288 = T1."Maximized" ("State")
            n98 = property class="VI"(reference=w294, error in=w293) -> (reference out=w291:refnum<vi>, error out=w292:errorcluster, "FP.State"=w290:T1)
            n99 = Not Equal?(x=w290, y=w288) -> (x != y?=w289:bool)
            n100 = case shown="True" w289 {
              tunnel: [w299 w300] -> w295
              tunnel: w292 -> [w298 w300]
              tunnel: w291 -> [w297 _]
              tunnel: w288 -> [w296 _]
              frame True {
                n101 = invoke class="VI" method="FP.Open"(reference=w297, error in=w298, "State"=w296) -> (error out=w299:errorcluster)  [unwired: 2 in, 4 out]
              }
              frame False {
              }
            }
          }
        }
      }
      frame "UI: Refresh Buttons" {
        # ":)"
        n102 = Unbundle By Name(w312) -> ("IsRunning?"=w302:bool)
        n103 = control-ref of="DAQ: Once"() -> (w311:refnum<vi>)
        n104 = control-ref of="Stop"() -> (w310:refnum<vi>)
        n105 = control-ref of="Start"() -> (w309:refnum<vi>)
        n106 = Not(x=w302) -> (.not. x?=w301:bool)
        n107 = Boolean To (0,1)(Boolean=w302) -> (0, 1=w308:i16)
        n108 = Boolean To (0,1)(Boolean=w301) -> (0, 1=w305:i16)
        n109 = Multiply(x=i16 2, y=w308) -> (x*y=w307:i16)
        n110 = Multiply(x=i16 2, y=w305) -> (x*y=w303:i16)
        n111 = property class="Bool"(reference=w311, "DisabledEnum"=w307) -> ()  [unwired: 1 in, 2 out]
        n112 = property class="Bool"(reference=w310, "DisabledEnum"=w303) -> ()  [unwired: 1 in, 2 out]
        n113 = property class="Bool"(reference=w309, "DisabledEnum"=w307) -> ()  [unwired: 1 in, 2 out]
      }
      frame "---------- Macro ----------" {
        # "#CSM \"Category Seperator\"\nDo not put any code in this frame."
        n114 = call <vilib>:"Add State(s) to Queue__JKI_lib_State_Machine.vi"("State(s) in (\"\")"=w318) -> ("States Out"=w317:string)  [unwired: 14 in]
      }
      frame "Macro: Initialize" {
        # "#CSM \"Macro: Initialize\"\nInitialization Macro (This is called once, when the VI starts)"
        n115 = call <vilib>:"Add State(s) to Queue__JKI_lib_State_Machine.vi"("State(s) in Front (\"\")"="Data: Initialize\nInitialize Core Data\nUI: Initialize\nData: Update Indicators", "State(s) in (\"\")"=w323) -> ("States Out"=w322:string)  [unwired: 13 in]
      }
      frame "Macro: DAQ Once" {
        n116 = call <vilib>:"Add State(s) to Queue__JKI_lib_State_Machine.vi"("State(s) in Front (\"\")"="DAQ: Initialize\nDAQ: Configure\nDAQ: Start\nData: Acquisite\nDAQ: Stop\nDAQ: Close\nUI: Refresh Buttons" ("State(s) in Front (\"\")"), "State(s) in (\"\")"=w325) -> ("States Out"=w326:string)  [unwired: 13 in]
      }
      frame "Macro: DAQ Continous" {
        n117 = call <vilib>:"Add State(s) to Queue__JKI_lib_State_Machine.vi"("State(s) in Front (\"\")"="DAQ: Initialize -><start>\nDAQ: Configure\nDAQ: Start\nUI: Refresh Buttons\nData: Acquisite\nDAQ: Continous Check -> <loop> \nDAQ: Stop\nDAQ: Close\nUI: Refresh Buttons -> <end>" ("State(s) in Front (\"\")"), "State(s) in (\"\")"=w330) -> ("States Out"=w331:string)  [unwired: 13 in]
      }
      frame "Macro: Exit" {
        # "#CSM \"Macro: Exit\"\nExit Macro (This is called once, when the VI exits)"
        n118 = call <vilib>:"Add State(s) to Queue__JKI_lib_State_Machine.vi"("State(s) in (\"\")"="//Exit Sub-Modules ", "State(s) at Back (\"\")"="Data: Cleanup\nExit") -> ("States Out"=w337:string)  [unwired: 13 in]
        n119 = call "CSM - Add Exit State(s) to Queue with Loop Check.vi"("States Out in"=w337, "Remaining States"=w334) -> ("States Out out"=w340:string)  [unwired: 13 in]
      }
      frame "---------- API ----------" {
        # "#CSM \"Category Seperator\"\nDo not put any code in this frame."
      }
      frame "API: API1" {
        # "#CSM API Example\nCopy/Rename this case for your own API"
        # "#CSM Response\nConnect this to return the response of your API"
        # "#CSM >> Source CSM >>\nIf you need to tell who triggered this state , use this string. If it's this case itself, this string is \"\"."
        # "#CSM >> Arguments >>\nDeal with the parameter if any"
      }
      frame "API: API2" {
        # "#CSM API Example\nCopy/Rename this case for your own API"
        # "unpack Hex String  to Variant\nif complex parameter is needed."
        n120 = call "CSM - Convert HexStr to Data.vi"("HEX String"=w349) -> ()  [unwired: 7 in, 2 out]
        n121 = disable-structure shown="Disabled" {
          disable-tunnel: [w353 "API2 Response"] -> w348
          frame Disabled {
            # "pack variant to hexstr \nif complex response is needed."
            # "complex Response"
            n122 = call "CSM - Convert Data to HexStr.vi"() -> ("HEX String (0-9,A-F)"=w353:string)  [unwired: 9 in]
          }
          frame Enabled {
          }
        }
      }
      frame "---------- Internal ----------" {
        # "#CSM \"Category Seperator\"\nDo not put any code in this frame."
        n123 = call <vilib>:"Add State(s) to Queue__JKI_lib_State_Machine.vi"("State(s) in (\"\")"=w358) -> ("States Out"=w357:string)  [unwired: 14 in]
      }
      frame "Internal: button click" {
        # "#CSM \"Internal State\"\nThis category is used for holding internal states"
        n124 = call <vilib>:"Add State(s) to Queue__JKI_lib_State_Machine.vi"("State(s) in (\"\")"=w362) -> ("States Out"=w361:string)  [unwired: 14 in]
      }
      frame "Internal: pane resize" {
        # "#CSM \"Internal State\"\nThis category is used for holding internal states"
        n125 = call <vilib>:"Add State(s) to Queue__JKI_lib_State_Machine.vi"("State(s) in (\"\")"=w366) -> ("States Out"=w365:string)  [unwired: 14 in]
      }
      frame "Internal: Slide Change" {
        n126 = Bundle By Name(cluster=w369, "Center"="Center") -> (w368:T4)
      }
      frame "----------- daq ---------------" {
      }
      frame "DAQ: Initialize" {
      }
      frame "DAQ: Configure" {
      }
      frame "DAQ: Start" {
        n127 = Bundle By Name(cluster=w383, "IsRunning?"=TRUE) -> (w382:T4)
      }
      frame "Data: Acquisite" {
        n128 = Unbundle By Name(w387) -> ("Center"=w386:dbl)
        n129 = Random Number (0-1)() -> (number: 0 to 1=w389:dbl)
        n130 = Add(x=w389, y=w386) -> (x+y=→"Waveform Chart":dbl)
      }
      frame "DAQ: Continous Check" {
        # "Loop timer"
        n131 = Wait (ms)(milliseconds to wait=u32 100) -> ()  [unwired: 1 out]
        n132 = call "CSM - Append Continious State.vi"("Loop State(s) and Arguments"="Data: Acquisite", "Continous Arguments (\"\")"=w393, "Continous State"=w394, "Remaining States"=w396) -> ("States Out"=w397:string)  [unwired: 7 in]
        ">> Source CSM >>" <- w395
      }
      frame "DAQ: Break Continous" {
        n133 = call "CSM - Remove Loop Tag to Break.vi"("Remaining States"=w402) -> ("States"=w401:string)  [unwired: 10 in]
      }
      frame "DAQ: Stop" {
        n134 = Bundle By Name(cluster=w407, "IsRunning?"=FALSE) -> (w406:T4)
      }
      frame "DAQ: Close" {
      }
    }
    "Remaining States" <- w66
  }
